vi "Read Cfg String.vi"(8 "error in (no error)":errorcluster, 11 "Get Serialized Device Configuration MSG in":refnum<class "Get Serialized Device Configuration MSG.lvclass">) -> (0 "error out":errorcluster, 2 "Cfg String":string, 3 "Get Serialized Device Configuration MSG out":refnum<class "Get Serialized Device Configuration MSG.lvclass">)   [LabVIEW 2014, in "Controller.lvlib" / "Get Serialized Device Configuration MSG.lvclass"]
uses:
  Get Serialized Device Configuration MSG.lvclass
  Get Serialized Device Configuration MSG.lvclass/Get Serialized Device Configuration MSG.ctl
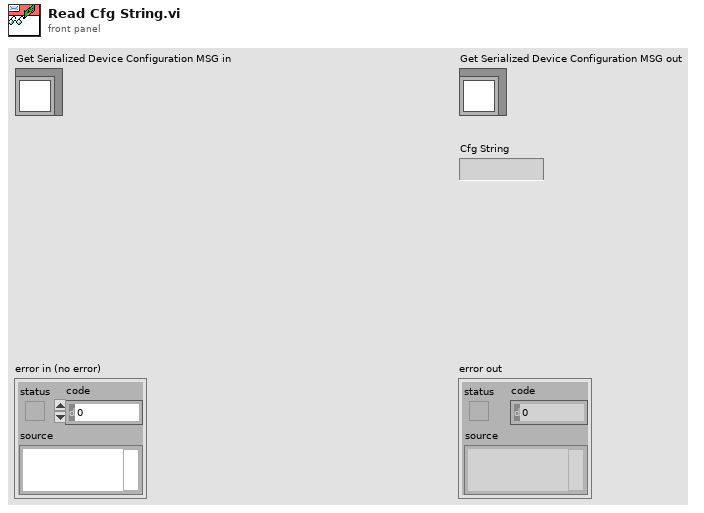
[diagram p1: front panel]
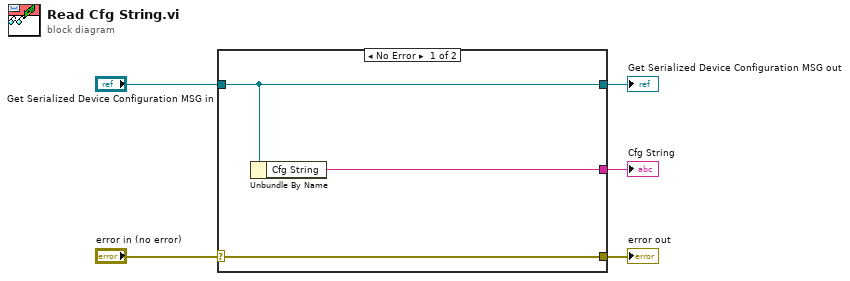
[diagram p0: block diagram]
diagram:
  n1 = case shown="No Error" "error in (no error)" {
    selector: "error in (no error)" -> [w8 w9]
    tunnel: [w8 w9] -> w4
    tunnel: [w7 w10] -> w2
    tunnel: "Get Serialized Device Configuration MSG in" -> [w7 w10]
    tunnel: [w6 _] -> w1
    frame No Error {
      n2 = Unbundle By Name(w7) -> ("Cfg String"=w6:string)
    }
    frame Error {
    }
  }
  "error out" <- w4
  "Get Serialized Device Configuration MSG out" <- w2
  "Cfg String" <- w1
